vi "FPGA.vi"() -> ()   [LabVIEW 2020]
uses:
  <vilib>/eio/EIONode/EIONode.xnode
  <vilib>/rvi/DataTransferAndStorage/Container/XNode/niFpgaContainer.xnode
  <vilib>/rvi/eio/common/nirviEmuTemplateMethod_errors.vi
  <vilib>/rvi/LocalResourceManager/LocalResourceManager.xnode
  <vilib>/rvi/FIFO/Fifo_Resource/niFpgaFifoEmulationRefIn.vi
  <vilib>/rvi/interface/RandomDataEmulation/nirviRandomDataFpgaReadWriteTemplate.vi
  <vilib>/Platform/TimedLoop/XDataNode/wakeup.ctl
  <vilib>/Platform/TimedLoop/XDataNode/XDNodeRunTimeDep.lvlib
  <vilib>/Platform/TimedLoop/XDataNode/nitl_modes.ctl
  <vilib>/Platform/TimedLoop/XDataNode/timing_clust.ctl
  <vilib>/platform/TimedLoop/XDataNode/XDataNode.xnode
  <vilib>/rvi/Analysis/measure/FFT/XNode/niFpgaFFT.xnode
  <vilib>/rvi/DataTransferAndStorage/Container/Common/niFpgaContainerGetUniqueNameForEmu.vi
  <vilib>/rvi/DataTransferAndStorage/Container/Common/niFpgaContainerSetEmuInfo.vi
  <vilib>/rvi/eio/common/nirviEmuReportErrorAndStop.vi
  <vilib>/rvi/FXPMathLib/FxpInterpret/XNode/nifxpmath_Interpret.xnode
  <vilib>/fxp/LVFixedPointQuantizationPolicyTypeDef.ctl
  <vilib>/rvi/Analysis/measure/FFT/simModelSupport/niFpgaFFTSimDfxp.ctl
  <vilib>/rvi/Analysis/measure/FFT/simModelSupport/niFpgaFFTSimArithmeticProperties.ctl
  <vilib>/rvi/Analysis/measure/FFT/simModelSupport/niFPGA FFT Sim Types.ctl
  <vilib>/rvi/Analysis/measure/FFT/simModelSupport/niFPGA FFT Sim Properties.ctl
  <vilib>/rvi/Analysis/measure/FFT/simModelSupport/niFpgaFFTSimModelCore.vi
panel:
  in  "FFT loop iterations":i32
  in  "auto stop":bool
  out "FFT time (uSec)":u32
  out "data collection time (uSec)":u32
  in  "Loop number":i32
  out "Element":fxp<+/-,24,7>
  out "Actual loop rate":u32
  in  "Rate (uSec)":u32 caption="Count(uSec)"
  out "Timed Out?":bool
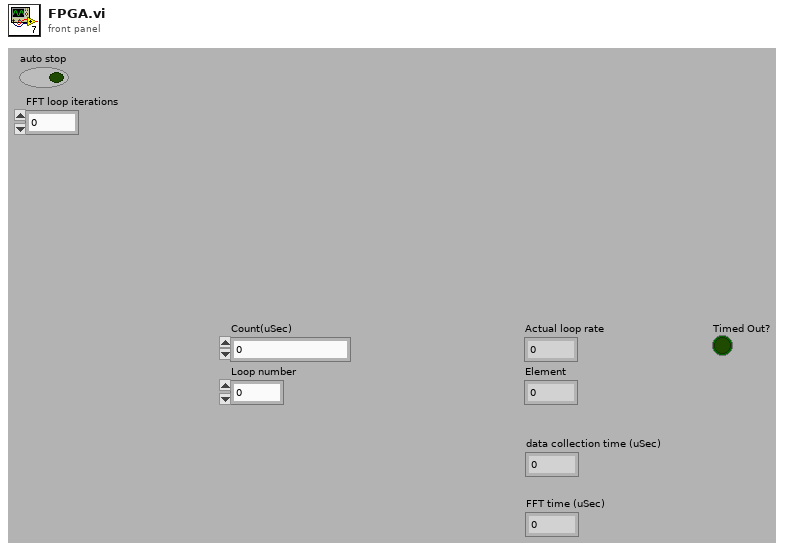
[diagram p1: front panel]
types:
  T1 = typedef "XDNodeRunTimeDep.lvlib/timing_clust.ctl" = cluster{"Expected End [f-1]":u64, "Actual End [f-1]":u64, "Finished Late? [f-1]":bool, "Expected End [i-1]":u64, "Actual End [i-1]":u64, "Finished Late? [i-1]":bool, "Expected Start [i]":u64, "Actual Start [i]":u64, "Expected Start [f]":u64, "Actual Start [f]":u64, "Source Name":string, "Structure Name":string, "Period":i64, "Deadline":i64, "Offset":i64, "Start":i64, "Priority":i32, "Timeout":i32, "Mode":T2, "Wakeup Reason":T3, "Error":errorcluster, "Source Type":string, "Secondary Source Type":string, "Global End Time":u64, "Global Start Time":u64, "Frame Duration":u64, "Iteration Duration":u64, "Assigned CPU":i32, "I/O Scan Engine Mode":u32}
  T2 = typedef "XDNodeRunTimeDep.lvlib/nitl_modes.ctl" = enum32{"No Change", "Process missed periods, maintain original phase", "Discard missed periods, maintain original phase", "Process missed periods, ignore original phase", "Discard missed periods, ignore original phase"}
  T3 = typedef "XDNodeRunTimeDep.lvlib/wakeup.ctl" = enum32{"Normal", "Aborted", "Asynchronous wakeup", "Timing source error", "Timed loop error", "Timeout"}
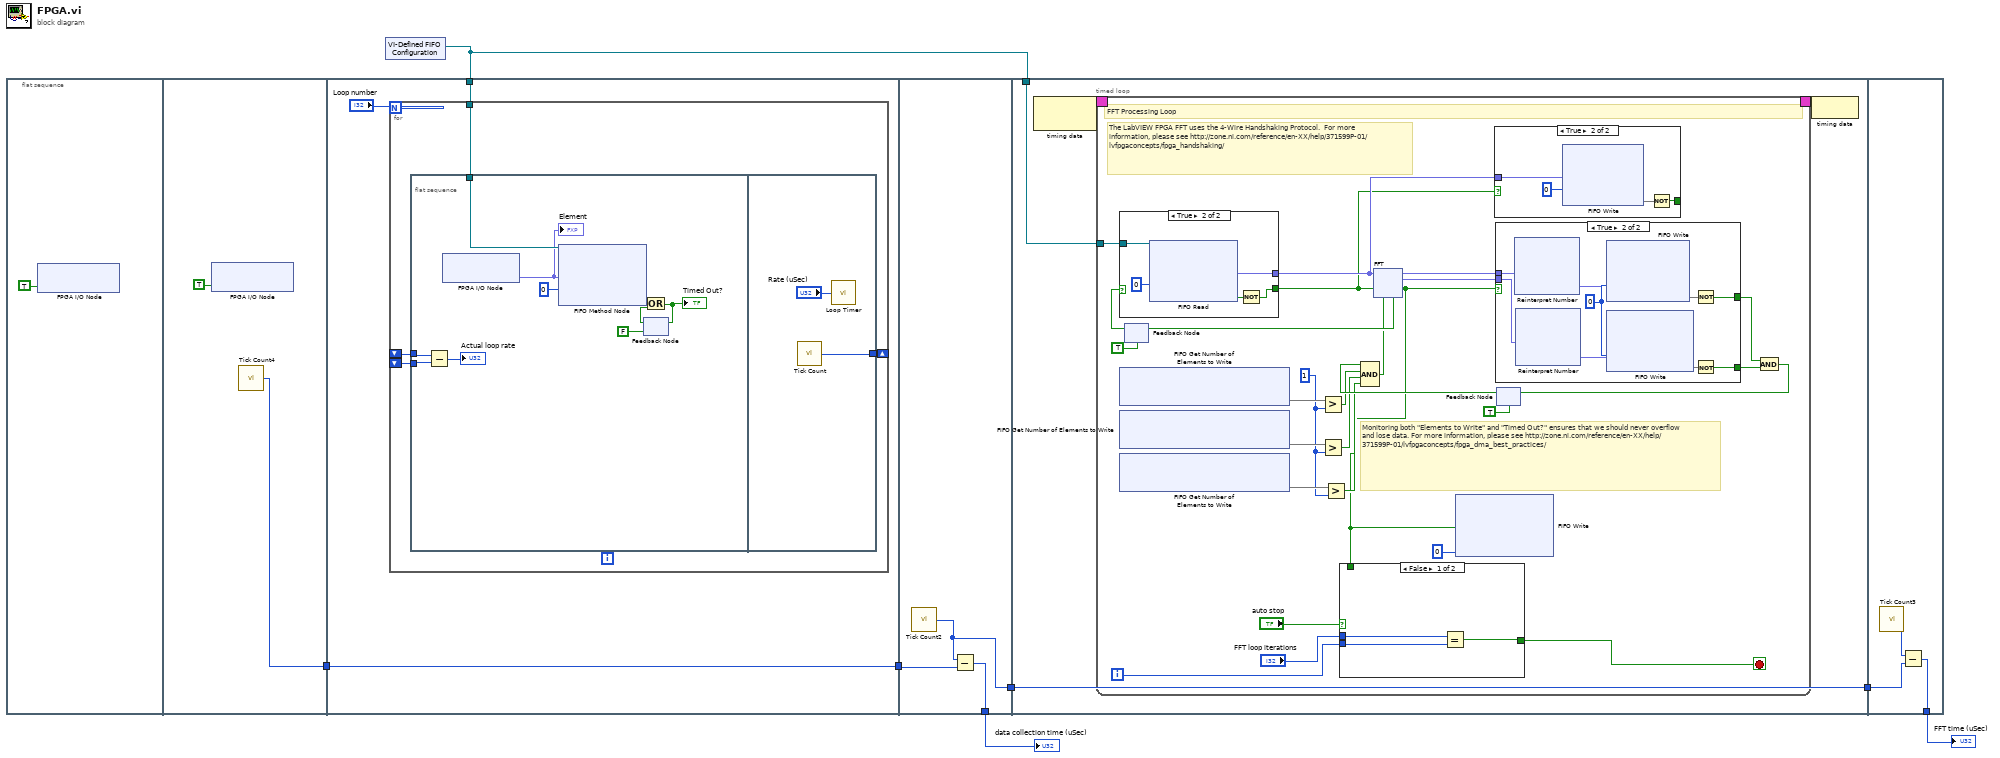
[diagram p0: block diagram]
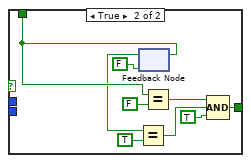
[diagram p2: hidden frame]
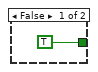
[diagram p3: hidden frame]
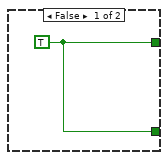
[diagram p4: hidden frame]
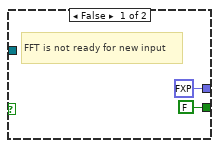
[diagram p5: hidden frame]
diagram:
  n1 = flat-sequence {
    tunnel: [w9] -> w6
    tunnel: w7 -> [w13]
    tunnel: w6 -> [w11]
    tunnel: [w11] -> w5
    tunnel: w5 -> [w32]
    tunnel: [w31] -> w4
    tunnel: [w30] -> w3
    tunnel: w7 -> [w34]
    tunnel: w3 -> [w33]
    tunnel: [w33] -> w2
    tunnel: w2 -> [w129]
    tunnel: [w128] -> w1
    frame #0 {
      n2 = xnode "FPGA I/O Node"("Mod1/Stop"=TRUE) -> ()  [unwired: 1 in, 1 out]
    }
    frame #1 {
      n3 = xnode "FPGA I/O Node"("Mod1/Start"=TRUE) -> ()  [unwired: 1 in, 1 out]
      n4 = call "Tick Count4"() -> ("Tick Count(uSec)"=w9:u32)
    }
    frame #2 {
      n5 = for {
        N: "Loop number" -> [_]
        shift-right: [w17] -> _
        shift-left: _ -> [w16]
        shift-left: _ -> [w15]
        tunnel: w13 -> [w14]
        n6 = flat-sequence {
          tunnel: w16 -> [w27]
          tunnel: w15 -> [w26]
          tunnel: w14 -> [w19]
          tunnel: [w28] -> w17
          frame #0 {
            n7 = Subtract(x=w27, y=w26) -> (x-y=→"Actual loop rate":u32)
            n8 = xnode "FPGA I/O Node"() -> ("Mod1/AI0"=w18:fxp<+/-,24,7>)  [unwired: 1 in, 1 out]
            "Element" <- w18
            n9 = xnode ("FIFO Method Node")("Element"=w18, "Timeout"=0, "FIFO In"=w19) -> ("Timed Out?"=w23:bool)  [unwired: 1 in, 2 out]
            n10 = feedback #1(FALSE) -> (w22:bool)
            n11 = Or(x=w23, y=w22) -> (x .or. y?=w21:bool)
            "Timed Out?" <- w21
            n12 = feedback-in #1(w21) -> ()
          }
          frame #1 {
            n13 = call "Tick Count"() -> ("Tick Count(uSec)"=w28:u32)
            n14 = call "Loop Timer"("Count(uSec)"="Rate (uSec)") -> ()  [unwired: 1 out]
          }
        }
      }
    }
    frame #3 {
      n15 = call "Tick Count2"() -> ("Tick Count(uSec)"=w30:u32)
      n16 = Subtract(x=w30, y=w32) -> (x-y=w31:u32)
    }
    frame #4 {
      n17 = node-c288() -> (w36:T1)  [unwired: 1 in]
      n18 = timed-loop {
        timing: w36 -> [_]
        timing-out: [_] -> w35
        tunnel: w34 -> [w60]
        i -> [w39]
        stop <- w42 stop-if-true
        w52 = u32 1 ("y")
        # "Monitoring both \"Elements to Write\" and \"Timed Out?\" ensures that we should never overflow and lose data. For more information, please see http://zone.ni.com/reference/en-XX/help/371599P-01/lvfpgaconcepts/fpga_dma_best_practices/"
        # "The LabVIEW FPGA FFT uses the 4-Wire Handshaking Protocol.  For more information, please see http://zone.ni.com/reference/en-XX/help/371599P-01/lvfpgaconcepts/fpga_handshaking/"
        # "FFT Processing Loop"
        n19 = xnode ("FIFO Get Number of Elements to Write")() -> ("Number of Elements to Write"=w55)  [unwired: 1 in, 1 out]
        n20 = xnode ("FIFO Get Number of Elements to Write")() -> ("Number of Elements to Write"=w54)  [unwired: 1 in, 1 out]
        n21 = xnode ("FIFO Get Number of Elements to Write")() -> ("Number of Elements to Write"=w53)  [unwired: 1 in, 1 out]
        n22 = feedback #2(TRUE ("ready for input")) -> (w63:bool)
        n23 = case shown="True" w63 {
          tunnel: [FALSE w122] -> w45
          tunnel: [fxp<+/-,16,5> 0.0 ("Element") w123] -> w62
          tunnel: w60 -> [_ w119]
          frame False {
            # "FFT is not ready for new input"
          }
          frame True {
            n24 = xnode ("FIFO Read")("Timeout"=0, "FIFO In"=w119) -> ("Element"=w123:fxp<+/-,24,7>, "Timed Out?"=w121:bool)  [unwired: 1 out]
            n25 = Not(x=w121) -> (.not. x?=w122:bool)
          }
        }
        n26 = Greater?(x=w55, y=w52) -> (0:w50:bool)
        n27 = Greater?(x=w54, y=w52) -> (0:w49:bool)
        n28 = Greater?(x=w53, y=w52) -> (0:w48:bool)
        n29 = case shown="True" w45 {
          tunnel: w62 -> [_ w77]
          tunnel: [TRUE ("Timed Out?") w78] -> _
          frame False {
          }
          frame True {
            n30 = xnode ("FIFO Write")("Element"=w77, "Timeout"=0) -> ("Timed Out?"=w79)  [unwired: 1 in, 1 out]
            n31 = Not(x=w79) -> (.not. x?=w78:bool)
          }
        }
        n32 = feedback #3(TRUE) -> (w51:bool)
        n33 = Compound Arithmetic op=AND(w51, w50, w49, w48) -> (w44:bool)
        n34 = xnode "FFT"("real data in"=w62, "input valid"=w45, "ready for output"=w44) -> ("ready for input"=w61:bool, "real data out"=w59:fxp<+/-,32,19>, "imaginary data out"=w41:fxp<+/-,32,19>, "output valid"=w37:bool)  [unwired: 2 in, 1 out]
        n35 = feedback-in #2(w61) -> ()
        n36 = case shown="False" "auto stop" {
          tunnel: w37 -> [_ w74]
          tunnel: [w64 w67] -> w42
          tunnel: w39 -> [w66 _]
          tunnel: "FFT loop iterations" -> [w65 _]
          frame False {
            n37 = Equal?(x=w65, y=w66) -> (x = y?=w64:bool)
          }
          frame True {
            n38 = feedback #4(FALSE) -> (w71:bool)
            n39 = Equal?(x=w71, y=TRUE) -> (x = y?=w69:bool)
            n40 = feedback-in #4(w74) -> ()
            n41 = Equal?(x=w74, y=FALSE) -> (x = y?=w70:bool)
            n42 = Compound Arithmetic op=AND(w70, w69, TRUE ("value")) -> (w67:bool)
          }
        }
        n43 = xnode ("FIFO Write")("Element"=w37, "Timeout"=0) -> ()  [unwired: 1 in, 2 out]
        n44 = case shown="True" w37 {
          tunnel: w59 -> [_ w111]
          tunnel: w41 -> [_ w109]
          tunnel: [w107 w113] -> w58
          tunnel: [w107 w112] -> w57
          frame False {
            w107 = TRUE ("Timed Out?")
          }
          frame True {
            w116 = 0 ("Timeout")
            n45 = xnode "Reinterpret Number"("x"=w111) -> ("y"=w110:fxp<+/-,32,21>)
            n46 = xnode "Reinterpret Number"("x"=w109) -> ("y"=w108:fxp<+/-,32,21>)
            n47 = xnode ("FIFO Write")("Element"=w110, "Timeout"=w116) -> ("Timed Out?"=w115)  [unwired: 1 in, 1 out]
            n48 = xnode ("FIFO Write")("Element"=w108, "Timeout"=w116) -> ("Timed Out?"=w114)  [unwired: 1 in, 1 out]
            n49 = Not(x=w115) -> (.not. x?=w113:bool)
            n50 = Not(x=w114) -> (.not. x?=w112:bool)
          }
        }
        n51 = Compound Arithmetic op=AND(w58, w57) -> (w46:bool)
        n52 = feedback-in #3(w46) -> ()
      }
      n53 = node-c288(w35) -> ()
    }
    frame #5 {
      n54 = call "Tick Count3"() -> ("Tick Count(uSec)"=w130:u32)
      n55 = Subtract(x=w130, y=w129) -> (x-y=w128:u32)
    }
  }
  n56 = xnode "VI-Defined FIFO Configuration"() -> ("FIFO Out"=w7:refnum<k21>)
  "data collection time (uSec)" <- w4
  "FFT time (uSec)" <- w1
